vi "GetParam.vi"(8 "error in (no error)":errorcluster caption="entrée d'erreur (pas d'erreur)", 11 "Brier_Score_Loss.lvclass":refnum<class "Brier_Score_Loss.lvclass">) -> (0 "error out":errorcluster caption="sortie d'erreur", 2 "brier_score_loss":T1={"sample_weight"=[], "pos_label"={"dtype_pos_label"="None", "pos_label"="None"}}, 3 "Brier_Score_Loss.lvclass":refnum<class "Brier_Score_Loss.lvclass">)   [LabVIEW 2020, in "Brier_Score_Loss.lvclass"]
doc: "Get Parameters"
uses:
  Brier_Score_Loss.lvclass
  Brier_Score_Loss.lvclass/Brier_Score_Loss.ctl
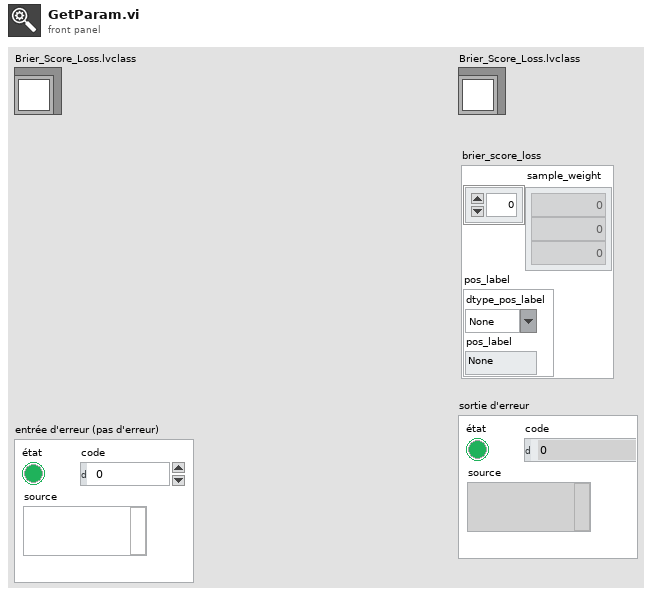
[diagram p1: front panel]
types:
  T1 = cluster{"sample_weight":dbl[], "pos_label":cluster{"dtype_pos_label":string, "pos_label":string}}
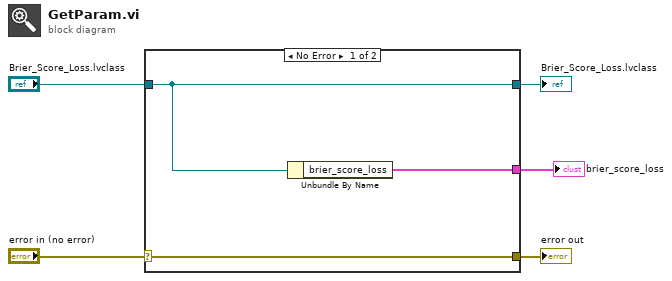
[diagram p0: block diagram]
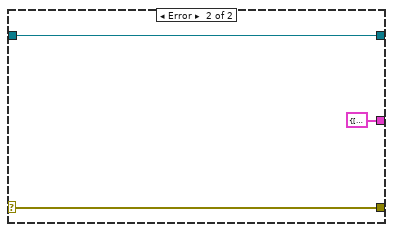
[diagram p2: hidden frame]
diagram:
  n1 = case shown="No Error" "error in (no error)" {
    selector: "error in (no error)" -> [w8 w10]
    tunnel: [w8 w10] -> w4
    tunnel: [w7 w11] -> w2
    tunnel: "Brier_Score_Loss.lvclass" -> [w7 w11]
    tunnel: [w6 T1 {"sample_weight"=[], "pos_label"={"dtype_pos_label"="", "pos_label"=""}} ("brier_score_loss")] -> w1
    frame No Error {
      n2 = Unbundle By Name(w7) -> ("brier_score_loss"=w6:T1)
    }
    frame Error {
    }
  }
  "error out" <- w4
  "Brier_Score_Loss.lvclass" <- w2
  "brier_score_loss" <- w1
